vi "CallChainRootName.vi"() -> (3 "VI Name":string)   [LabVIEW 2019]
uses:
  TextToVariant.vi
  BlueJSONTextSerializer.lvclass
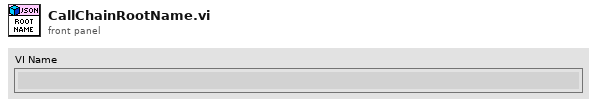
[diagram p1: front panel]
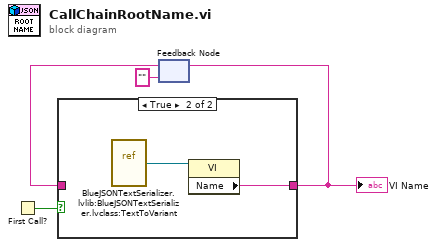
[diagram p0: block diagram]
diagram:
  n1 = First Call?() -> (First Call?: T/F=w4:bool)
  n2 = feedback #1("" ("Name")) -> (w1:string)
  n3 = case shown="True" w4 {
    tunnel: [w5 w6] -> w3
    tunnel: w1 -> [w5 _]
    frame False {
    }
    frame True {
      n4 = vi-ref "BlueJSONTextSerializer.lvlib:BlueJSONTextSerializer.lvclass:TextToVariant.vi"() -> (w7:refnum<vi>)
      n5 = property class="VI"(reference=w7) -> ("Name"=w6:string)  [unwired: 1 in, 2 out]
    }
  }
  "VI Name" <- w3
  n6 = feedback-in #1(w3) -> ()
